vi "Robotics Environment Simulator.vi"() -> ()   [LabVIEW 2015]
doc: "This VI starts and stops the environment simulator and serves as the master VI for your simulation code. Open and run this VI to display the environment simulator, or open the block diagram to view or modify simulation code."
uses:
  <vilib>/Platform/TimedLoop/XDataNode/timing_clust.ctl
  <vilib>/Platform/TimedLoop/XDataNode/nitl_modes.ctl
  <vilib>/Platform/TimedLoop/XDataNode/wakeup.ctl
  <vilib>/Utility/AngleManip/Degrees to Radians (Scalar DBL).vi
  <vilib>/imath/engines/lvmath2/RunTimeEngine/IndexReplace/NIMS M(S,$)=V.vi
  <instcachedir>/0/NIMS M(S,$)=V_260679A9E30142119AFD27BBD2C5FD93.lvgen/NIMS M(S,$)=V_260679A9E30142119AFD27BBD2C5FD93_002.vi
  <vilib>/imathl/engines/lvmath/Functions/Error Handling/Create Error.vi
  <vilib>/imath/engines/lvmath2/RunTimeEngine/IndexReplace/NIMS M(S,S)=S.vi
  <instcachedir>/0/NIMS M(S,S)=S_72298AC072A24B679F5E0C14DB2DD503.lvgen/NIMS M(S,S)=S_72298AC072A24B679F5E0C14DB2DD503_002.vi
  <vilib>/imath/engines/lvmath2/RunTimeEngine/RangeToken/NIMS_Range_R2 - Integer.vi
  <instcachedir>/0/NIMS_Range_R2 - Integer_396D5D4FB869421F9245109A0975AD54.lvgen/NIMS_Range_R2 - Integer_396D5D4FB869421F9245109A0975AD54_000.vi
  <vilib>/imath/engines/lvmath2/RunTimeEngine/CommandStatement/MC_CommandStatement_break.vi
  <vilib>/imath/engines/lvmath2/RunTimeEngine/BuiltInFunctions/mod/NIMS_mod_no_size_check.vi
  <instcachedir>/0/NIMS_mod_no_size_check_5393E3382FD241D281EEB71DA286C65B.lvgen/NIMS_mod_no_size_check_5393E3382FD241D281EEB71DA286C65B_001.vi
  <vilib>/imath/engines/lvmath2/RunTimeEngine/VariableToken/NIMS_VariableToken_CondDefinedDefinedByReplace.vi
  <instcachedir>/0/NIMS_VariableToken_CondDefinedDefinedByReplace_D162CFFC24174562A9FEA619A91E1A56.lvgen/NIMS_VariableToken_CondDefinedDefinedByReplace_D162CFFC24174562A9FEA619A91E1A56_001.vi
  <instcachedir>/0/NIMS M(S,S)=S_72298AC072A24B679F5E0C14DB2DD503.lvgen/NIMS M(S,S)=S_72298AC072A24B679F5E0C14DB2DD503_000.vi
  <vilib>/imath/engines/lvmath2/RunTimeEngine/IndexRead/NIMS M(S,S).vi
  <instcachedir>/0/NIMS M(S,S)_AC51E74150A542F7991B9634C66F3096.lvgen/NIMS M(S,S)_AC51E74150A542F7991B9634C66F3096_000.vi
  <vilib>/imath/engines/lvmath2/RunTimeSupport/NIMS_Error if Not Equal.vi
  <instcachedir>/0/NIMS_Error if Not Equal_7F0D61CE56BF44979916ECA34C78675F.lvgen/NIMS_Error if Not Equal_7F0D61CE56BF44979916ECA34C78675F_000.vi
  <instcachedir>/0/NIMS M(S,S)_AC51E74150A542F7991B9634C66F3096.lvgen/NIMS M(S,S)_AC51E74150A542F7991B9634C66F3096_002.vi
  <vilib>/imath/engines/lvmath2/RunTimeEngine/ErrorHandling/NIMS_Create Error From Enums.vi
  <vilib>/imath/engines/lvmath2/RunTimeEngine/CommandStatement/NIMS_CommandStatement_MaskErr.vi
  <vilib>/imath/engines/lvmath2/RunTimeEngine/VariableToken/NIMS_VariableToken_CondDefined.vi
  <instcachedir>/0/NIMS_VariableToken_CondDefined_FE30D0A1BFB24F098D41DEBABFE96BE1.lvgen/NIMS_VariableToken_CondDefined_FE30D0A1BFB24F098D41DEBABFE96BE1_001.vi
  <vilib>/imath/engines/lvmath2/RunTimeEngine/IndexRead/NIMS M(S,$).vi
  <instcachedir>/0/NIMS M(S,$)_F24F360562DE41D8BE234322A2E15C65.lvgen/NIMS M(S,$)_F24F360562DE41D8BE234322A2E15C65_000.vi
  Documents/LabVIEW Data/MathScriptVIs/MCStatic_35241984432_878391c453101b8ea8a3a082d24a9a1b.vi
  <instcachedir>/0/MCStatic_35241984432_878391c453101b8ea8a3a082d24a9a1b_1C0BCF58ECF54AF19A642F074C09ACBC.lvgen/MCStatic_35241984432_878391c453101b8ea8a3a082d24a9a1b_1C0BCF58ECF54AF19A642F074C09ACBC_000.vi
  <vilib>/imath/engines/lvmath/Functions/Error Handling/MergeErrorsWrapper.vi
  <vilib>/imath/engines/lvmath2/RunTimeEngine/NodeEndStatement/NIMS_NodeEndStatement_Output.vi
  <instcachedir>/0/NIMS_NodeEndStatement_Output_53EC0D466D134D7ABD903AC30B43404B.lvgen/NIMS_NodeEndStatement_Output_53EC0D466D134D7ABD903AC30B43404B_012.vi
  <instcachedir>/0/NIMS_NodeEndStatement_Output_53EC0D466D134D7ABD903AC30B43404B.lvgen/NIMS_NodeEndStatement_Output_53EC0D466D134D7ABD903AC30B43404B_010.vi
  <instcachedir>/0/NIMS_NodeEndStatement_Output_53EC0D466D134D7ABD903AC30B43404B.lvgen/NIMS_NodeEndStatement_Output_53EC0D466D134D7ABD903AC30B43404B_002.vi
  <vilib>/imath/engines/lvmath2/RunTimeEngine/ErrorHandling/NIMS_Finalize Error.vi
  <vilib>/robotics/Steering/Steering Frame/Apply Steering Frame Velocity to Motors.vi
  <instcachedir>/0/NIMS_VariableToken_CondDefined_FE30D0A1BFB24F098D41DEBABFE96BE1.lvgen/NIMS_VariableToken_CondDefined_FE30D0A1BFB24F098D41DEBABFE96BE1_004.vi
  <instcachedir>/0/NIMS_NodeEndStatement_Output_53EC0D466D134D7ABD903AC30B43404B.lvgen/NIMS_NodeEndStatement_Output_53EC0D466D134D7ABD903AC30B43404B_005.vi
  <instcachedir>/0/NIMS_NodeEndStatement_Output_53EC0D466D134D7ABD903AC30B43404B.lvgen/NIMS_NodeEndStatement_Output_53EC0D466D134D7ABD903AC30B43404B_013.vi
  <instcachedir>/0/NIMS_NodeEndStatement_Output_53EC0D466D134D7ABD903AC30B43404B.lvgen/NIMS_NodeEndStatement_Output_53EC0D466D134D7ABD903AC30B43404B_001.vi
  <vilib>/imath/engines/lvmath2/RunTimeEngine/Managers/WorkSpace/UID Generator.vi
  <vilib>/imath/engines/lvmath2/RunTimeEngine/IndexRead/NIMS M($,S).vi
  <instcachedir>/0/NIMS M($,S)_3E5749BBB62E49528D4765A77F1F6D98.lvgen/NIMS M($,S)_3E5749BBB62E49528D4765A77F1F6D98_000.vi
  <vilib>/imath/engines/lvmath2/RunTimeEngine/RunTimeType/NIMS_RunTimeType_From StrictType (excl LVString).vi
  <instcachedir>/0/NIMS_RunTimeType_From StrictType (excl LVString)_EB1C38A9BC5048DA9ABDA8F781E54D21.lvgen/NIMS_RunTimeType_From StrictType (excl LVString)_EB1C38A9BC5048DA9ABDA8F781E54D21_000.vi
  <vilib>/imath/engines/lvmath2/RunTimeEngine/LocalVariableDefStatement/MC_LocalVariableDefStatement_Display.vi
  <vilib>/imath/engines/lvmath2/RunTimeEngine/Managers/SymbolTable/Clear UID.vi
  <vilib>/Platform/TimedLoop/XDataNode/XDataNode.xnode
  Documents/LabVIEW Data/eatbean2.m
  <vilib>/robotics/Starter Kit/2.0/Sim Host Interface/NI_Robotics_Starter Kit Host_Sim_2.0.lvclass
  <vilib>/robotics/Simulator/NI_Robotics_Simulator.lvlib
  <vilib>/Platform/TimedLoop/XDataNode/XDNodeRunTimeDep.lvlib
  <vilib>/robotics/Steering/Steering Frame/NI_Robotics_Steering Frame.lvclass
  <vilib>/robotics/Starter Kit/Host Interface/NI_Robotics_Starter Kit Host.lvclass
  <vilib>/robotics/Utilities/Scan Angles/NI_Robotics_Scan Angles.lvlib
  <vilib>/Utility/AngleManip/NI_AngleManipulation.lvlib
  <vilib>/robotics/Starter Kit/2.0/NI_Robotics_Starter Kit Host_2.0.lvlib
  <vilib>/imath/engines/lvmath2/RunTimeEngine/Managers/SymbolTable/NIMS_WorkSpace.lvlib
panel:
  out "a":dbl[](array[numeric])
  out "b":dbl[](array[numeric])
  out "XY Graph":cluster{"xi":dbl[], "yi":dbl[]}[](graph)
  out "bean":dbl[][](array[numeric])
  in  "stop 3":bool
  out "Sensor Data 2":cluster{"angles (deg)":dbl[], "distances":dbl[]}(graph)
  out "new_angle 2":dbl
  out "new_x 2":dbl
  out "new_y 2":dbl
  out "distances 2":dbl[](array[numeric])
  out "angles 2":dbl[](array[numeric])
  out "v1_next 2":dbl
  out "v2_next 2":dbl
  out "left motor ccw velocity (rad/s) 2":dbl
  out "right motor ccw velocity (rad/s) 2":dbl
  out "headDest":dbl[](array[numeric])
  out "headIndex":i64
  out "headDirect":i32
  in  "stop 2":bool
  out "Sensor Data":cluster{"angles (deg)":dbl[], "distances":dbl[]}(graph)
  out "new_angle":dbl
  out "new_x":dbl
  out "new_y":dbl
  out "distances":dbl[](array[numeric])
  out "angles":dbl[](array[numeric])
  out "v1_next":dbl
  out "v2_next":dbl
  out "left motor ccw velocity (rad/s)":dbl
  out "right motor ccw velocity (rad/s)":dbl
  out "tailIndex":i64
  out "tailDest":dbl[](array[numeric])
  out "tailMoveto":i32
  out "tailDirect":i32
  in  "manifest filename":string="Robotics Environment Simulator.xml"
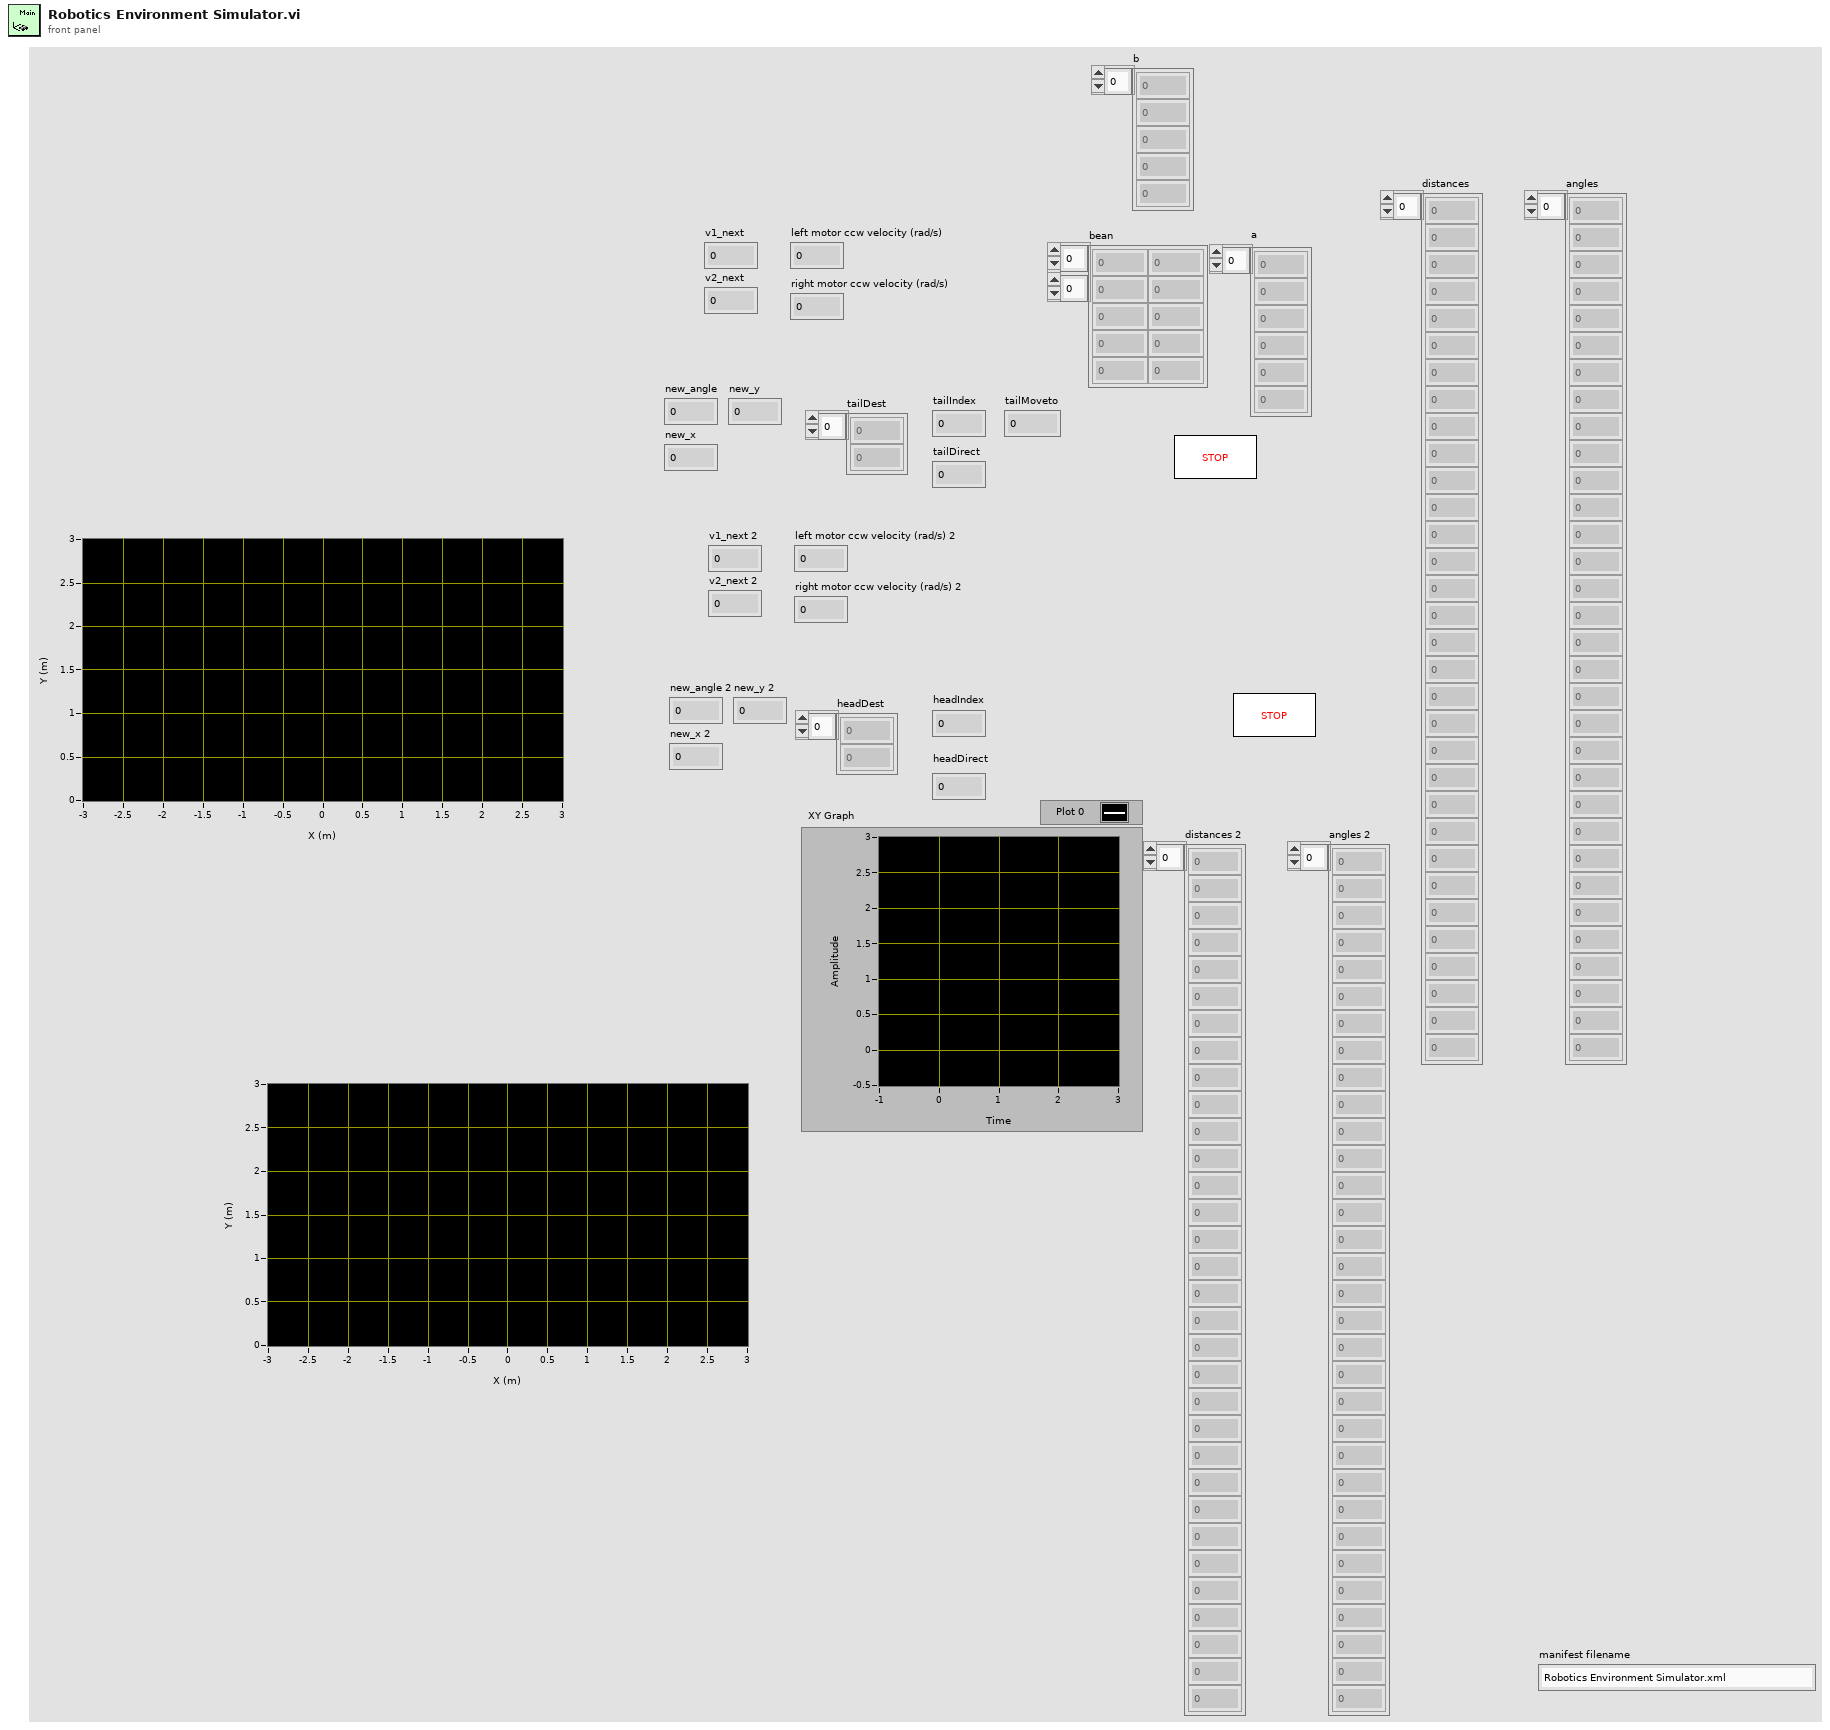
[diagram p1: front panel]
types:
  T1 = typedef "NI_Robotics_Scan Angles.lvlib/Scan Angle Data.ctl" = cluster{"angles":dbl[], "distances":dbl[], "current index":i32, "previous index":i32}
  T2 = typedef "XDNodeRunTimeDep.lvlib/timing_clust.ctl" = cluster{"Expected End [f-1]":u64, "Actual End [f-1]":u64, "Finished Late? [f-1]":bool, "Expected End [i-1]":u64, "Actual End [i-1]":u64, "Finished Late? [i-1]":bool, "Expected Start [i]":u64, "Actual Start [i]":u64, "Expected Start [f]":u64, "Actual Start [f]":u64, "Source Name":string, "Structure Name":string, "Period":i64, "Deadline":i64, "Offset":i64, "Start":i64, "Priority":i32, "Timeout":i32, "Mode":T3, "Wakeup Reason":T4, "Error":errorcluster, "Source Type":string, "Secondary Source Type":string, "Global End Time":u64, "Global Start Time":u64, "Frame Duration":u64, "Iteration Duration":u64, "Assigned CPU":i32, "I/O Scan Engine Mode":u32}
  T3 = typedef "XDNodeRunTimeDep.lvlib/nitl_modes.ctl" = enum32{"No Change", "Process missed periods, maintain original phase", "Discard missed periods, maintain original phase", "Process missed periods, ignore original phase", "Discard missed periods, ignore original phase"}
  T4 = typedef "XDNodeRunTimeDep.lvlib/wakeup.ctl" = enum32{"Normal", "Aborted", "Asynchronous wakeup", "Timing source error", "Timed loop error", "Timeout"}
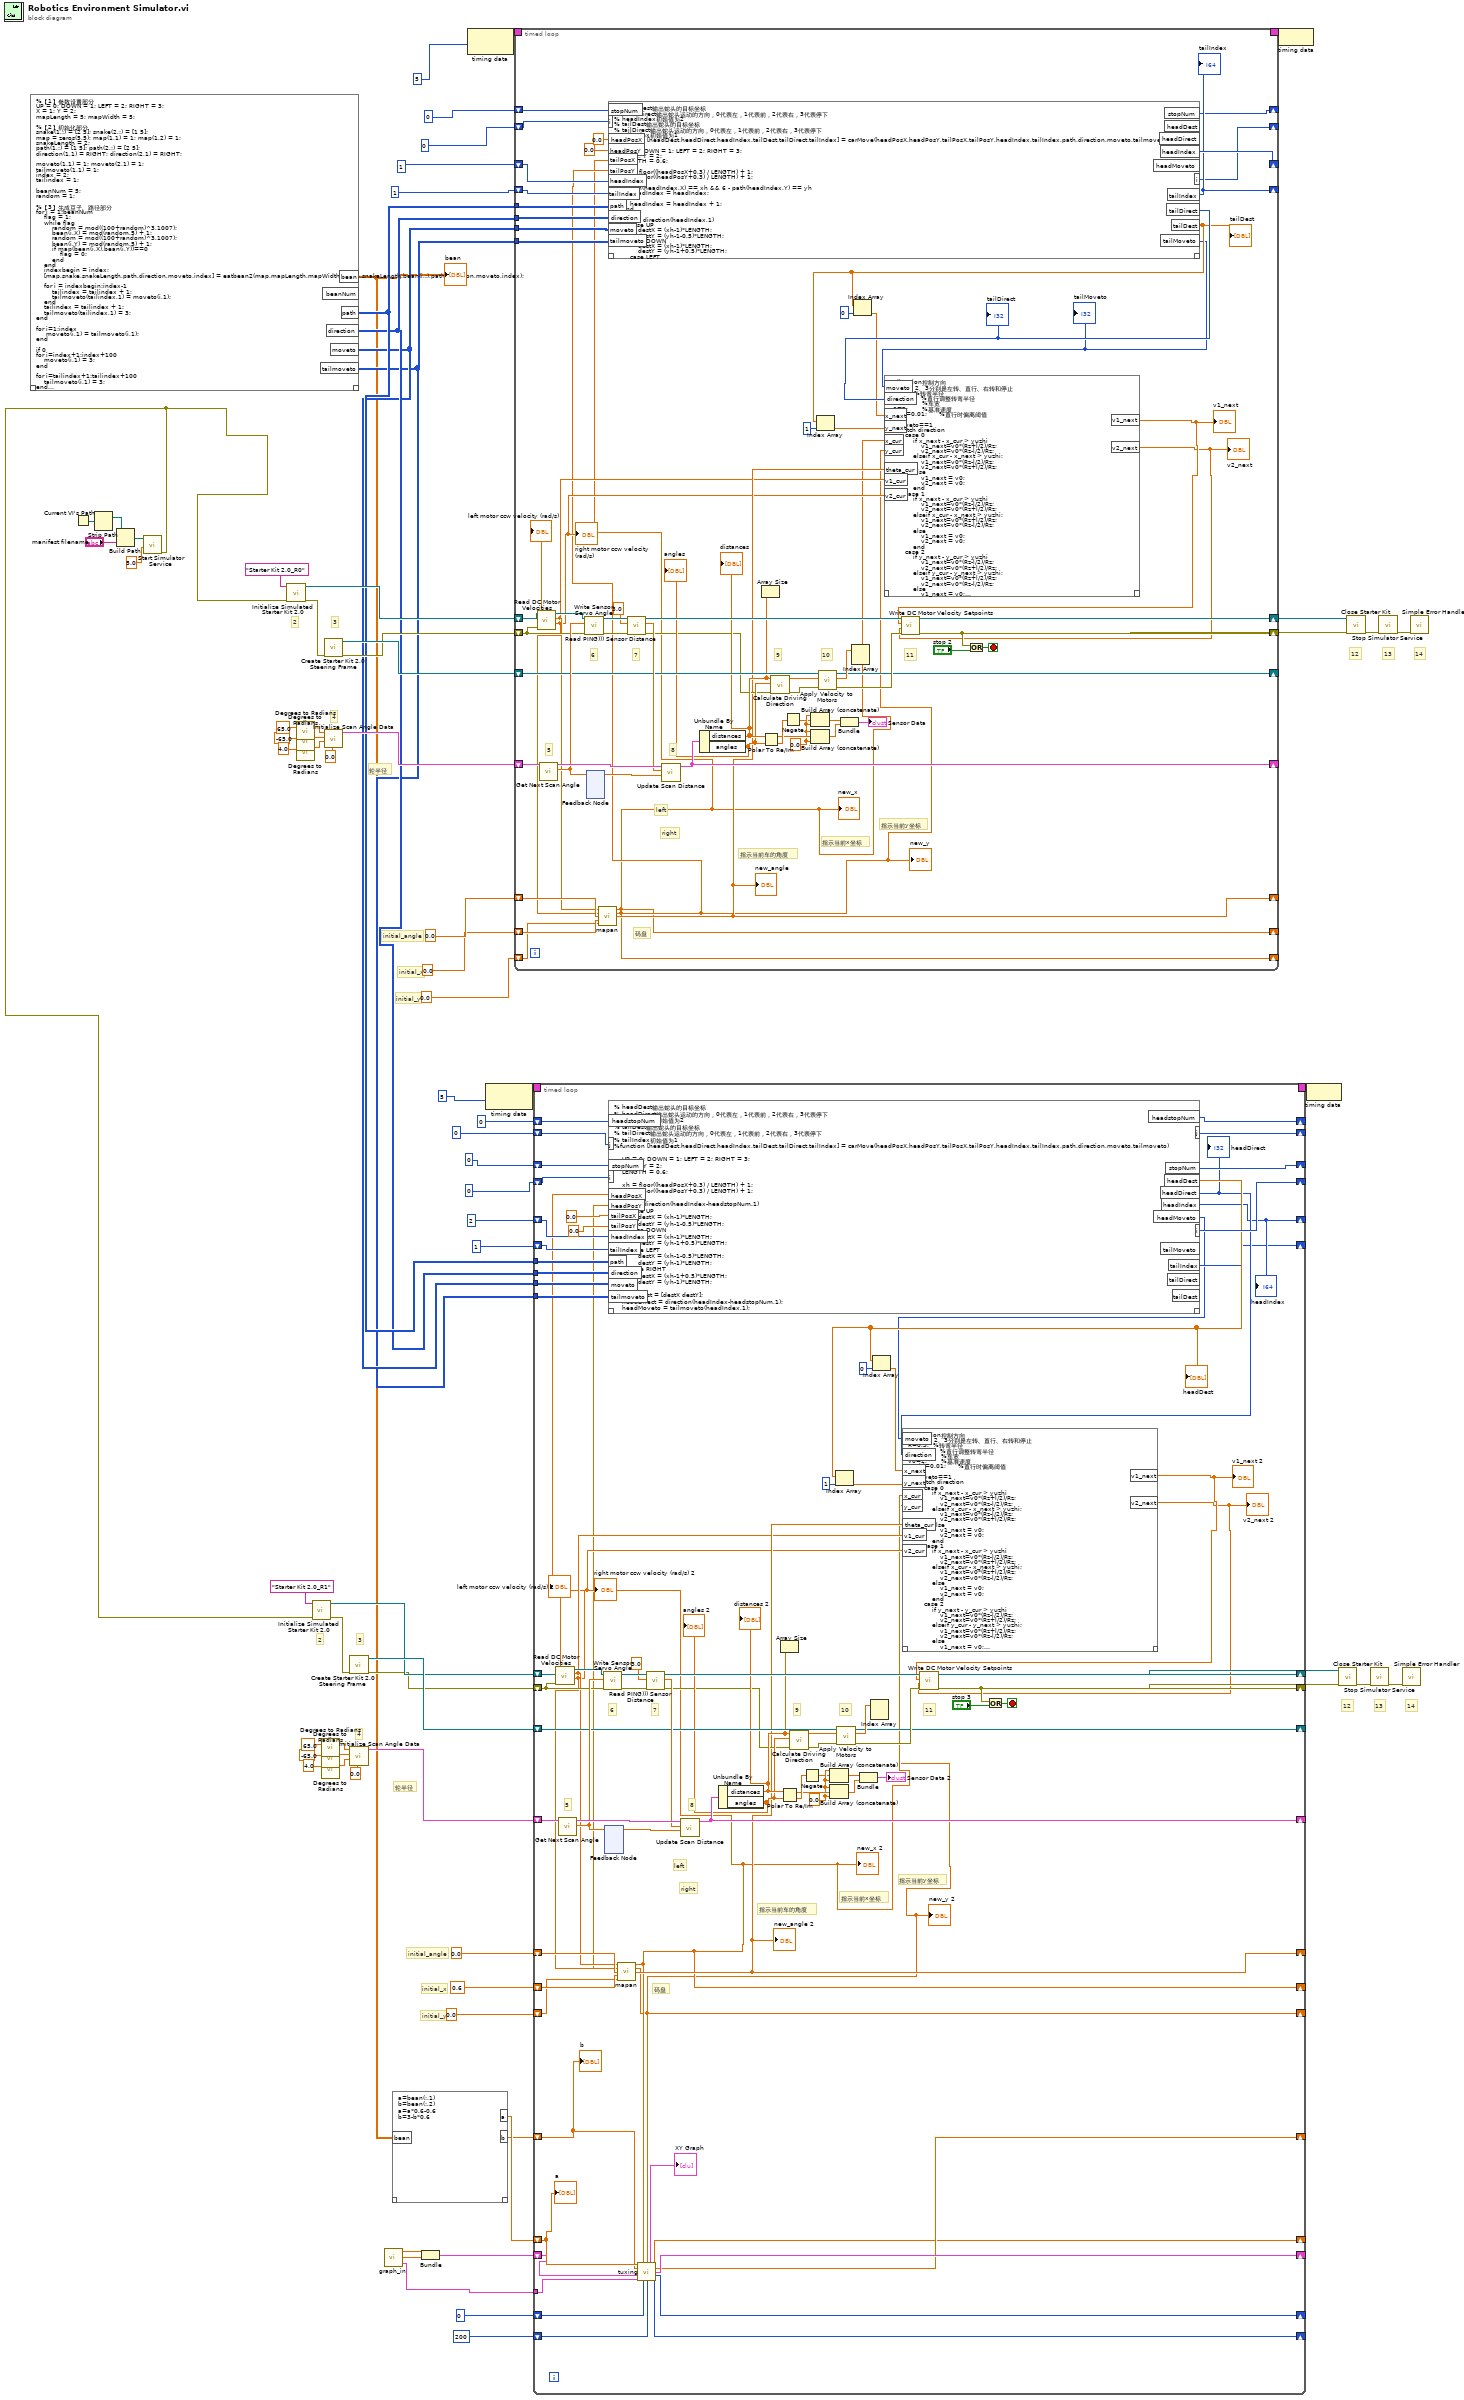
[diagram p0: block diagram]
diagram:
  # "initial_x"
  # "轮半径"
  # "initial_y"
  # "initial_angle"
  # "14"
  # "13"
  # "12"
  # "2"
  # "3"
  # "4"
  # "轮半径"
  # "initial_y"
  # "initial_x"
  # "initial_angle"
  # "14"
  # "13"
  # "12"
  # "2"
  # "3"
  # "4"
  n1 = mathscript code="%【1】参数设置部分\nUP = 0; DOWN = 1; LEFT = 2; RIGHT = 3;\nX = 1; Y = 2;\nmapLength = 5; mapWidth = 5;\n\n%【2】初始化部分\nsnake(1,:) = [2 5]; snake(2,:) = [1 5];\nmap = zeros(5,5); map(1,1) = 1; map(1,2) = 1;\nsnakeLength = 2;\npath(1,:) = [1 5]; path(2,:) = [2 5];\ndirection(1,1) = RIGHT; direction(2,1) = RIGHT;\n    \nmoveto(1,1) = 1; moveto(2,1) = 1;\ntailmoveto(1,1) = 1;\nindex = 2;\ntailindex = 1;\n    \nbeanNum = 5;\nrandom = 1;\n\n%【3】生成豆子、路径部分\nfor i = 1:beanNum\n    flag = 1;\n    while flag\n        random = mod((100+random)^3,1007);\n        bean(i,X) = mod(random,5) + 1;\n        random = mod((100+random)^3,1007);\n        bean(i,Y) = mod(random,5) + 1;\n        if map(bean(i,X),bean(i,Y))==0\n            flag = 0;\n        end\n    end\n    indexbegin = index;\n    [map,snake,snakeLength,path,direction,moveto,index] = eatbean2(map,mapLength,mapWidth,snake,snakeLength,bean(i,:),path,direction,moveto,index);\n    \n    for i = indexbegin:index-1\n        tailindex = tailindex + 1;\n        tailmoveto(tailindex,1) = moveto(i,1);\n    end\n    tailindex = tailindex + 1;\n    tailmoveto(tailindex,1) = 3;\nend\n\nfor i=1:index\n     moveto(i,1) = tailmoveto(i,1);\nend\n\nif 0\nfor i=index+1:index+100\n    moveto(i,1) = 3;\nend\n\nfor i=tailindex+1:tailindex+100\n    tailmoveto(i,1) = 3;\nend\nend"() -> ("bean"=w9:dbl[][], "path"=w16:i32[][], "direction"=w15:i32[][], "moveto"=w14:i32[][], "tailmoveto"=w13:i32[][])  [unwired: 1 in, 2 out]
  "bean" <- w9
  n2 = Current VI's Path() -> (path=w74:path)
  n3 = Strip Path(path=w74) -> (stripped path=w73:path)  [unwired: 1 out]
  n4 = Build Path(base path=w73, name or relative path="manifest filename") -> (appended path=w72:path)
  n5 = call <vilib>:"Start Simulator Service.vi"("step size (ms)"=5.0 ("stepsize(ms)"), "manifest file"=w72) -> ("error out"=w10:errorcluster)  [unwired: 9 in]
  n6 = call <vilib>:"Initialize Simulated Starter Kit 2.0.vi"("error in (no error)"=w10, "robot ID"="Starter Kit 2.0_R0") -> ("error out"=w64:errorcluster, "simulated starter kit host 2.0 out"=w65:refnum<class "NI_Robotics_Starter Kit Host_Sim_2.0.lvclass">)  [unwired: 8 in]
  n7 = call-poly <vilib>:"Degrees to Radians.vi"("angle (deg)"=65.0 ("max angle")) -> ("angle (rad)"=w60:dbl)  [unwired: 2 in]
  n8 = call-poly <vilib>:"Degrees to Radians.vi"("angle (deg)"=-65.0 ("min angle")) -> ("angle (rad)"=w56:dbl)  [unwired: 2 in]
  n9 = call-poly <vilib>:"Degrees to Radians.vi"("angle (deg)"=4.0 ("scan angle")) -> ("angle (rad)"=w57:dbl)  [unwired: 2 in]
  n10 = call <vilib>:"Initialize Simulated Starter Kit 2.0.vi"("error in (no error)"=w10, "robot ID"="Starter Kit 2.0_R1") -> ("error out"=w39:errorcluster, "simulated starter kit host 2.0 out"=w40:refnum<class "NI_Robotics_Starter Kit Host_Sim_2.0.lvclass">)  [unwired: 8 in]
  n11 = call-poly <vilib>:"Degrees to Radians.vi"("angle (deg)"=65.0 ("max angle")) -> ("angle (rad)"=w35:dbl)  [unwired: 2 in]
  n12 = call-poly <vilib>:"Degrees to Radians.vi"("angle (deg)"=-65.0 ("min angle")) -> ("angle (rad)"=w31:dbl)  [unwired: 2 in]
  n13 = call-poly <vilib>:"Degrees to Radians.vi"("angle (deg)"=4.0 ("scan angle")) -> ("angle (rad)"=w32:dbl)  [unwired: 2 in]
  n14 = call <vilib>:"Create Starter Kit 2.0 Steering Frame.vi"("error in (no error)"=w64) -> ("error out"=w54:errorcluster, "starter kit differential steering frame"=w66:refnum<class "NI_Robotics_Differential Steering Frame.lvclass">)  [unwired: 9 in]
  n15 = call <vilib>:"Initialize Scan Angle Data.vi"("initial angle (0)"=0.0, "scan angle"=w57, "min angle"=w56, "max angle"=w60) -> ("scan angles"=w55:T1)  [unwired: 6 in, 1 out]
  n16 = call <vilib>:"Create Starter Kit 2.0 Steering Frame.vi"("error in (no error)"=w39) -> ("error out"=w29:errorcluster, "starter kit differential steering frame"=w41:refnum<class "NI_Robotics_Differential Steering Frame.lvclass">)  [unwired: 9 in]
  n17 = call <vilib>:"Initialize Scan Angle Data.vi"("initial angle (0)"=0.0, "scan angle"=w32, "min angle"=w31, "max angle"=w35) -> ("scan angles"=w30:T1)  [unwired: 6 in, 1 out]
  n18 = call "graph_in.vi"() -> ("map"=w3:cluster{"x":dbl[], "y":dbl[]}, "y0"=w5:dbl[], "x0"=w6:dbl[])
  n19 = mathscript code="a=bean(:,1)\nb=bean(:,2)\na=a*0.6-0.6\nb=3-b*0.6"("bean"=w9) -> ("a"=w8:dbl[], "b"=w7:dbl[])  [unwired: 1 in, 1 out]
  n20 = Bundle("x0"=w6, "y0"=w5) -> (w4:cluster{"x0":dbl[], "y0":dbl[]})  [unwired: 1 in]
  n21 = node-c288(i64 5 ("Period")) -> (w70:T2)
  n22 = node-c288(i64 5 ("Period")) -> (w68:T2)
  n23 = timed-loop {
    shift-right: [w124] -> w63
    shift-left: w65 -> [w111]
    shift-right: [w113] -> w62
    shift-left: w54 -> [w112]
    shift-right: [w126] -> _
    shift-left: w66 -> [w127]
    timing: w70 -> [_]
    timing-out: [_] -> w69
    shift-right: [w123] -> _
    shift-left: w55 -> [w128]
    shift-right: [w103] -> _
    shift-left: 0.0 -> [w106]
    shift-right: [w89] -> _
    shift-left: 0.0 -> [w105]
    shift-right: [w90] -> _
    shift-left: 0.0 -> [w104]
    tunnel: w16 -> [w100]
    tunnel: w15 -> [w97]
    tunnel: w14 -> [w99]
    tunnel: w13 -> [w98]
    shift-right: [w95] -> _
    shift-left: i64 1 ("Period") -> [w96]
    shift-right: [w94] -> _
    shift-left: i64 1 ("Period") -> [w93]
    shift-right: [w83] -> _
    shift-left: i64 0 ("Period") -> [w84]
    shift-right: [w81] -> _
    shift-left: i64 0 ("Period") -> [w82]
    stop <- w125 stop-if-true
    w119 = 0.0 ("element")
    # "指示当前y坐标"
    # "指示当前x坐标"
    # "指示当前车的角度"
    # "码盘"
    # "right"
    # "left"
    # "7"
    # "6"
    # "11"
    # "10"
    # "9"
    # "8"
    # "5"
    n24 = call <vilib>:"Read DC Motor Velocities.vi"("error in (no error)"=w112, "starter kit host in"=w111) -> ("right motor ccw velocity (rad/s)"=w101:dbl, "left motor ccw velocity (rad/s)"=w102:dbl, "starter kit host out"=w110:refnum<class "NI_Robotics_Starter Kit Host_Sim_2.0.lvclass">)  [unwired: 6 in, 1 out]
    "left motor ccw velocity (rad/s)" <- w102
    "right motor ccw velocity (rad/s)" <- w101
    n25 = call <vilib>:"Get Next Scan Angle.vi"("scan angles in"=w128) -> ("new angle"=w135:dbl, "scan angles out"=w138:T1)  [unwired: 9 in]
    n26 = call <vilib>:"Write Sensor Servo Angle.vi"("error in (no error)"=w112, "ccw servo angle (rad)"=w135, "starter kit host in"=w110) -> ("error out"=w132:errorcluster, "starter kit host out"=w133:refnum<class "NI_Robotics_Starter Kit Host_Sim_2.0.lvclass">)  [unwired: 7 in]
    n27 = feedback #1() -> (w137:dbl)  [unwired: 1 in]
    n28 = feedback-in #1(w135) -> ()
    n29 = call "mapan.vi"("lwf"=w102, "rwf"=w101, "direct"=w106, "xposit"=w105, "yposit"=w104) -> ("xposit 2"=w89:dbl, "yposit 2"=w90:dbl, "direct 2"=w103:dbl)  [unwired: 8 in]
    "new_angle" <- w103
    "new_x" <- w89
    "new_y" <- w90
    n30 = mathscript code="% headDest输出蛇头的目标坐标\n% headDirect输出蛇头运动的方向，0代表左，1代表前，2代表右，3代表停下\n% headIndex初始值为2\n% tailDest输出蛇头的目标坐标\n% tailDirect输出蛇头运动的方向，0代表左，1代表前，2代表右，3代表停下\n% tailIndex初始值为1\n%function [headDest,headDirect,headIndex,tailDest,tailDirect,tailIndex] = carMove(headPosX,headPosY,tailPosX,tailPosY,headIndex,tailIndex,path,direction,moveto,tailmoveto)\n\nUP = 0; DOWN = 1; LEFT = 2; RIGHT = 3;\n    X = 1; Y = 2;\n    LENGTH = 0.6;\n    \n    xh = floor((headPosX+0.3) / LENGTH) + 1;\n    yh = floor((headPosY+0.3) / LENGTH) + 1;\n    \n    if path(headIndex,X) == xh && 6 - path(headIndex,Y) == yh\n        headIndex = headIndex;\n    else\n        headIndex = headIndex + 1;\n    end\n    \n    switch direction(headIndex,1)\n        case UP\n            destX = (xh-1)*LENGTH;\n            destY = (yh-1-0.5)*LENGTH;\n        case DOWN\n            destX = (xh-1)*LENGTH;\n            destY = (yh-1+0.5)*LENGTH;\n        case LEFT\n            destX = (xh-1-0.5)*LENGTH;\n            destY = (yh-1)*LENGTH;\n        case RIGHT\n            destX = (xh-1+0.5)*LENGTH;\n            destY = (yh-1)*LENGTH;\n    end\n    headDest = [destX destY];\n    headDirect = direction(headIndex,1);\n    headMoveto = moveto(headIndex,1);\n    \n    xt = floor((tailPosX+0.3) / LENGTH) + 1;\n    yt = floor((tailPosY+0.3) / LENGTH) + 1;\n\n    switch direction(tailIndex-stopNum,1)\n        case UP\n            destX = (xt-1)*LENGTH;\n            destY = (yt-1-0.5)*LENGTH;\n        case DOWN\n            destX = (xt-1)*LENGTH;\n            destY = (yt-1+0.5)*LENGTH;\n        case LEFT\n            destX = (xt-1-0.5)*LENGTH;\n            destY = (yt-1)*LENGTH;\n        case RIGHT\n            destX = (xt-1+0.5)*LENGTH;\n            destY = (yt-1)*LENGTH;\n    end\n    tailDest = [destX destY];\n    tailDirect = direction(tailIndex-stopNum,1);\n    tailMoveto = tailmoveto(tailIndex,1);\n\n    if tailMoveto==3\n        if i<1200\n            i = i + 1;\n            tailIndex = tailIndex;\n        else\n            i = 0;\n            tailIndex = tailIndex + 1;\n            stopNum = stopNum + 1;\n        end\n    elseif path(tailIndex-stopNum,X) == xt && (6 - path(tailIndex-stopNum,Y) == yt)\n        tailIndex = tailIndex;\n    else\n        tailIndex = tailIndex + 1;\n    end"("headPosX"=0.0, "headPosY"=0.0, "tailPosX"=w89, "tailPosY"=w90, "headIndex"=w96, "tailIndex"=w93, "path"=w100, "direction"=w97, "moveto"=w99, "tailmoveto"=w98, "i"=w84, "stopNum"=w82) -> ("headIndex"=w95:i64, "tailIndex"=w94:i64, "tailDirect"=w88:i32, "tailDest"=w87:dbl[], "i"=w83:i64, "stopNum"=w81:i64, "tailMoveto"=w76:i32)  [unwired: 1 in, 4 out]
    "tailIndex" <- w94
    "tailDest" <- w87
    "tailMoveto" <- w76
    "tailDirect" <- w88
    n31 = call <vilib>:"Read PING))) Sensor Distance.vi"("error in (no error)"=w132, "default distance (NaN)"=3.0, "starter kit host in"=w133) -> ("error out"=w107:errorcluster, "distance (m)"=w134:dbl, "starter kit host out"=w131:refnum<class "NI_Robotics_Starter Kit Host_Sim_2.0.lvclass">)  [unwired: 5 in, 1 out]
    n32 = call <vilib>:"Update Scan Distance.vi"("scan angle"=w137, "new scan distance"=w134, "scan angles in"=w138) -> ("scan angles out"=w123:T1)  [unwired: 8 in]
    n33 = Unbundle By Name(w123) -> ("distances"=w109:dbl[], "angles"=w108:dbl[])
    "distances" <- w109
    "angles" <- w108
    n34 = Array Size(array=w109) -> ()  [unwired: 1 out]
    n35 = Polar To Re/Im(2:w108, 3:w109) -> (0:w122:dbl[], 1:w121:dbl[])
    n36 = call "Calculate Driving Direction.vi"("error in (no error)"=w107, "obstacle angles (rad)"=w108, "obstacle distances (m)"=w109) -> ("error out"=w114:errorcluster, "steering frame velocity"=w115:dbl[])  [unwired: 7 in]
    n37 = Negate(x=w122) -> (-x=w117:dbl[])
    n38 = Build Array (concatenate)(w119, w117, w119) -> (w118:dbl[])
    n39 = Build Array (concatenate)(w119, w121, w119) -> (w120:dbl[])
    n40 = Index Array(array=w87, index=1) -> (element=w79:dbl)
    n41 = call-poly <vilib>:"Apply Velocity to Motors.vi"("error in (no error)"=w114, "steering frame velocity"=w115, "steering frame in"=w127) -> ("error out"=w130:errorcluster, "ccw motor velocity setpoints"=w136:dbl[], "steering frame out"=w126:refnum<class "NI_Robotics_Differential Steering Frame.lvclass">)  [unwired: 4 in, 2 out]
    n42 = Bundle(w118, w120) -> (→"Sensor Data":cluster{dbl[], dbl[]})  [unwired: 1 in]
    n43 = Index Array(array=w136) -> ()  [unwired: 2 in, 2 out]
    n44 = Index Array(array=w87, index=0) -> (element=w80:dbl)
    n45 = mathscript code="%direction控制方向\n%0、1、2、3分别是左转、直行、右转和停止\nR=0.3;  %转弯半径\nRz=1.5;    %直行调整转弯半径\nl=0.36;     %车宽\nv0=2;       %基准速度\nyuzhi=0.01;      %直行时偏离阈值\n\nif moveto==1\n    switch direction\n        case 0\n            if x_next - x_cur > yuzhi\n                v1_next=v0*(Rz+l/2)/Rz;\n                v2_next=v0*(Rz-l/2)/Rz;\n            elseif x_cur - x_next > yuzhi;\n                v1_next=v0*(Rz-l/2)/Rz;\n                v2_next=v0*(Rz+l/2)/Rz;\n            else\n                v1_next = v0;\n                v2_next = v0;\n            end\n        case 1\n            if x_next - x_cur > yuzhi\n                v1_next=v0*(Rz-l/2)/Rz;\n                v2_next=v0*(Rz+l/2)/Rz;\n            elseif x_cur - x_next > yuzhi;\n                v1_next=v0*(Rz+l/2)/Rz;\n                v2_next=v0*(Rz-l/2)/Rz;\n            else\n                v1_next = v0;\n                v2_next = v0;\n            end\n        case 2\n            if y_next - y_cur > yuzhi\n                v1_next=v0*(Rz-l/2)/Rz;\n                v2_next=v0*(Rz+l/2)/Rz;\n            elseif y_cur - y_next > yuzhi;\n                v1_next=v0*(Rz+l/2)/Rz;\n                v2_next=v0*(Rz-l/2)/Rz;\n            else\n                v1_next = v0;\n                v2_next = v0;\n            end\n        case 3\n            if y_next - y_cur > yuzhi\n                v1_next=v0*(Rz+l/2)/Rz;\n                v2_next=v0*(Rz-l/2)/Rz;\n            elseif y_cur - y_next > yuzhi;\n                v1_next=v0*(Rz-l/2)/Rz;\n                v2_next=v0*(Rz+l/2)/Rz;\n            else\n                v1_next = v0;\n                v2_next = v0;\n            end\n    end\nelseif moveto==0\n    v1_next=v0*(R-l/2)/R;\n    v2_next=v0*(R+l/2)/R;\nelseif moveto==2\n    v1_next=v0*(R+l/2)/R;\n    v2_next=v0*(R-l/2)/R;\nelse\n    if v1_cur>0.8 && v2_cur>0.8\n        v1_next=v1_cur-0.5;\n        v2_next=v2_cur-0.5;\n    else\n        v1_next=0;\n        v2_next=0;\n    end\nend\nv2_next=-v2_next;"("x_next"=w80, "y_next"=w79, "x_cur"=w89, "y_cur"=w90, "theta_cur"=w103, "v1_cur"=w102, "v2_cur"=w101, "direction"=w88, "moveto"=w76) -> ("v1_next"=w78:dbl, "v2_next"=w77:dbl)  [unwired: 1 in, 1 out]
    "v1_next" <- w78
    "v2_next" <- w77
    n46 = call <vilib>:"Write DC Motor Velocity Setpoints.vi"("error in (no error)"=w130, "right motor ccw velocity (rad/s)"=w77, "left motor ccw velocity (rad/s)"=w78, "starter kit host in"=w131) -> ("error out"=w113:errorcluster, "starter kit host out"=w124:refnum<class "NI_Robotics_Starter Kit Host_Sim_2.0.lvclass">)  [unwired: 6 in]
    n47 = Or(x=w113, y="stop 2") -> (x .or. y?=w125:bool)
  }
  n48 = timed-loop {
    shift-right: [w1967] -> w38
    shift-left: w40 -> [w1954]
    shift-right: [w1956] -> w37
    shift-left: w29 -> [w1955]
    shift-right: [w1969] -> _
    shift-left: w41 -> [w1970]
    timing: w68 -> [_]
    timing-out: [_] -> w67
    shift-right: [w1966] -> _
    shift-left: w30 -> [w1971]
    shift-right: [w1946] -> _
    shift-left: 0.0 -> [w1949]
    shift-right: [w1909] -> _
    shift-left: 0.6 -> [w1948]
    shift-right: [w1908] -> _
    shift-left: 0.0 -> [w1947]
    tunnel: w16 -> [w1943]
    tunnel: w15 -> [w1940]
    tunnel: w14 -> [w1942]
    tunnel: w13 -> [w1941]
    shift-right: [w1923] -> _
    shift-left: i64 2 ("Period") -> [w1939]
    shift-right: [w1922] -> _
    shift-left: i64 1 ("Period") -> [w1938]
    shift-right: [w1934] -> _
    shift-left: i64 0 ("Period") -> [w1935]
    shift-right: [w1932] -> _
    shift-left: i64 0 ("Period") -> [w1933]
    shift-right: [w1918] -> _
    shift-left: i64 0 ("Period") -> [w1920]
    shift-right: [w1917] -> _
    shift-left: i64 0 ("Period") -> [w1919]
    tunnel: w3 -> [w1913]
    shift-right: [w1907] -> _
    shift-left: 0 -> [w1912]
    shift-right: [w1906] -> _
    shift-left: 200 -> [w1911]
    shift-right: [w1903] -> _
    shift-left: w8 -> [w1916]
    shift-right: [w1904] -> _
    shift-left: w7 -> [w1915]
    shift-right: [w1905] -> _
    shift-left: w4 -> [w1914]
    stop <- w1968 stop-if-true
    w1962 = 0.0 ("element")
    # "指示当前y坐标"
    # "指示当前x坐标"
    # "指示当前车的角度"
    # "码盘"
    # "right"
    # "left"
    # "7"
    # "6"
    # "11"
    # "10"
    # "9"
    # "8"
    # "5"
    n49 = call <vilib>:"Read DC Motor Velocities.vi"("error in (no error)"=w1955, "starter kit host in"=w1954) -> ("right motor ccw velocity (rad/s)"=w1944:dbl, "left motor ccw velocity (rad/s)"=w1945:dbl, "starter kit host out"=w1953:refnum<class "NI_Robotics_Starter Kit Host_Sim_2.0.lvclass">)  [unwired: 6 in, 1 out]
    "left motor ccw velocity (rad/s) 2" <- w1945
    "right motor ccw velocity (rad/s) 2" <- w1944
    n50 = call <vilib>:"Get Next Scan Angle.vi"("scan angles in"=w1971) -> ("new angle"=w1978:dbl, "scan angles out"=w1981:T1)  [unwired: 9 in]
    n51 = call <vilib>:"Write Sensor Servo Angle.vi"("error in (no error)"=w1955, "ccw servo angle (rad)"=w1978, "starter kit host in"=w1953) -> ("error out"=w1975:errorcluster, "starter kit host out"=w1976:refnum<class "NI_Robotics_Starter Kit Host_Sim_2.0.lvclass">)  [unwired: 7 in]
    n52 = feedback #2() -> (w1980:dbl)  [unwired: 1 in]
    n53 = feedback-in #2(w1978) -> ()
    n54 = call "mapan.vi"("lwf"=w1945, "rwf"=w1944, "direct"=w1949, "xposit"=w1948, "yposit"=w1947) -> ("xposit 2"=w1909:dbl, "yposit 2"=w1908:dbl, "direct 2"=w1946:dbl)  [unwired: 8 in]
    "new_angle 2" <- w1946
    "new_x 2" <- w1909
    "new_y 2" <- w1908
    n55 = mathscript code="% headDest输出蛇头的目标坐标\n% headDirect输出蛇头运动的方向，0代表左，1代表前，2代表右，3代表停下\n% headIndex初始值为2\n% tailDest输出蛇头的目标坐标\n% tailDirect输出蛇头运动的方向，0代表左，1代表前，2代表右，3代表停下\n% tailIndex初始值为1\n%function [headDest,headDirect,headIndex,tailDest,tailDirect,tailIndex] = carMove(headPosX,headPosY,tailPosX,tailPosY,headIndex,tailIndex,path,direction,moveto,tailmoveto)\n\n    UP = 0; DOWN = 1; LEFT = 2; RIGHT = 3;\n    X = 1; Y = 2;\n    LENGTH = 0.6;\n    \n    xh = floor((headPosX+0.3) / LENGTH) + 1;\n    yh = floor((headPosY+0.3) / LENGTH) + 1;\n    \n    switch direction(headIndex-headstopNum,1)\n        case UP\n            destX = (xh-1)*LENGTH;\n            destY = (yh-1-0.5)*LENGTH;\n        case DOWN\n            destX = (xh-1)*LENGTH;\n            destY = (yh-1+0.5)*LENGTH;\n        case LEFT\n            destX = (xh-1-0.5)*LENGTH;\n            destY = (yh-1)*LENGTH;\n        case RIGHT\n            destX = (xh-1+0.5)*LENGTH;\n            destY = (yh-1)*LENGTH;\n    end\n    headDest = [destX destY];\n    headDirect = direction(headIndex-headstopNum,1);\n    headMoveto = tailmoveto(headIndex,1);\n    \n    if headMoveto==3\n        if j<150\n            j = j + 1;\n            headIndex = headIndex;\n        else\n            j = 0;\n            headIndex = headIndex + 1;\n            headstopNum = headstopNum + 1;\n        end\n    elseif path(headIndex-headstopNum,X) == xh && (6 - path(headIndex-headstopNum,Y) == yh)\n        headIndex = headIndex;\n    else\n        headIndex = headIndex + 1;\n    end\n\n    xt = floor((tailPosX+0.3) / LENGTH) + 1;\n    yt = floor((tailPosY+0.3) / LENGTH) + 1;\n\n    switch direction(tailIndex-stopNum,1)\n        case UP\n            destX = (xt-1)*LENGTH;\n            destY = (yt-1-0.5)*LENGTH;\n        case DOWN\n            destX = (xt-1)*LENGTH;\n            destY = (yt-1+0.5)*LENGTH;\n        case LEFT\n            destX = (xt-1-0.5)*LENGTH;\n            destY = (yt-1)*LENGTH;\n        case RIGHT\n            destX = (xt-1+0.5)*LENGTH;\n            destY = (yt-1)*LENGTH;\n    end\n    tailDest = [destX destY];\n    tailDirect = direction(tailIndex-stopNum,1);\n    tailMoveto = tailmoveto(tailIndex,1);\n\n    if tailMoveto==3\n        if i<1200\n            i = i + 1;\n            tailIndex = tailIndex;\n        else\n            i = 0;\n            tailIndex = tailIndex + 1;\n            stopNum = stopNum + 1;\n        end\n    elseif path(tailIndex-stopNum,X) == xt && (6 - path(tailIndex-stopNum,Y) == yt)\n        tailIndex = tailIndex;\n    else\n        tailIndex = tailIndex + 1;\n    end"("headPosX"=w1909, "headPosY"=w1908, "tailPosX"=0.0, "tailPosY"=0.0 ("tailPosX"), "headIndex"=w1939, "tailIndex"=w1938, "path"=w1943, "direction"=w1940, "moveto"=w1942, "tailmoveto"=w1941, "i"=w1935, "stopNum"=w1933, "j"=w1920, "headstopNum"=w1919) -> ("headIndex"=w1923:i64, "tailIndex"=w1922:i64, "headDirect"=w1927:i32, "headDest"=w1929:dbl[], "i"=w1934:i64, "stopNum"=w1932:i64, "headMoveto"=w1921:i32, "j"=w1918:i64, "headstopNum"=w1917:i64)  [unwired: 1 in, 4 out]
    "headDest" <- w1929
    "headIndex" <- w1923
    "headDirect" <- w1927
    n56 = call "tuxing.vi"("bean_x"=w1916, "xnew"=w1909, "ynew"=w1908, "bean_y"=w1915, "xy_in"=w1914, "map_in"=w1913, "n1"=w1912, "n2"=w1911) -> ("XY Graph"=→"XY Graph":cluster{"xi":dbl[], "yi":dbl[]}[], "a"=w1903:dbl[], "b"=w1904:dbl[], "pos_o"=w1905:cluster{"xo":dbl[], "yo":dbl[]}, "n1 2"=w1907:i32, "n2 2"=w1906:i32)  [unwired: 2 in]
    n57 = call <vilib>:"Read PING))) Sensor Distance.vi"("error in (no error)"=w1975, "default distance (NaN)"=3.0, "starter kit host in"=w1976) -> ("error out"=w1950:errorcluster, "distance (m)"=w1977:dbl, "starter kit host out"=w1974:refnum<class "NI_Robotics_Starter Kit Host_Sim_2.0.lvclass">)  [unwired: 5 in, 1 out]
    n58 = call <vilib>:"Update Scan Distance.vi"("scan angle"=w1980, "new scan distance"=w1977, "scan angles in"=w1981) -> ("scan angles out"=w1966:T1)  [unwired: 8 in]
    n59 = Unbundle By Name(w1966) -> ("distances"=w1952:dbl[], "angles"=w1951:dbl[])
    "distances 2" <- w1952
    "angles 2" <- w1951
    n60 = Array Size(array=w1952) -> ()  [unwired: 1 out]
    n61 = Polar To Re/Im(2:w1951, 3:w1952) -> (0:w1965:dbl[], 1:w1964:dbl[])
    n62 = call "Calculate Driving Direction.vi"("error in (no error)"=w1950, "obstacle angles (rad)"=w1951, "obstacle distances (m)"=w1952) -> ("error out"=w1957:errorcluster, "steering frame velocity"=w1958:dbl[])  [unwired: 7 in]
    n63 = Negate(x=w1965) -> (-x=w1960:dbl[])
    n64 = Build Array (concatenate)(w1962, w1960, w1962) -> (w1961:dbl[])
    n65 = Build Array (concatenate)(w1962, w1964, w1962) -> (w1963:dbl[])
    n66 = Index Array(array=w1929, index=1) -> (element=w1930:dbl)
    n67 = call-poly <vilib>:"Apply Velocity to Motors.vi"("error in (no error)"=w1957, "steering frame velocity"=w1958, "steering frame in"=w1970) -> ("error out"=w1973:errorcluster, "ccw motor velocity setpoints"=w1979:dbl[], "steering frame out"=w1969:refnum<class "NI_Robotics_Differential Steering Frame.lvclass">)  [unwired: 4 in, 2 out]
    n68 = Bundle(w1961, w1963) -> (→"Sensor Data 2":cluster{dbl[], dbl[]})  [unwired: 1 in]
    n69 = Index Array(array=w1979) -> ()  [unwired: 2 in, 2 out]
    n70 = Index Array(array=w1929, index=0) -> (element=w1931:dbl)
    n71 = mathscript code="%direction控制方向\n%0、1、2、3分别是左转、直行、右转和停止\nR=0.3;  %转弯半径\nRz=1.5;    %直行调整转弯半径\nl=0.36;     %车宽\nv0=2;       %基准速度\nyuzhi=0.01;      %直行时偏离阈值\n\nif moveto==1\n    switch direction\n        case 0\n            if x_next - x_cur > yuzhi\n                v1_next=v0*(Rz+l/2)/Rz;\n                v2_next=v0*(Rz-l/2)/Rz;\n            elseif x_cur - x_next > yuzhi;\n                v1_next=v0*(Rz-l/2)/Rz;\n                v2_next=v0*(Rz+l/2)/Rz;\n            else\n                v1_next = v0;\n                v2_next = v0;\n            end\n        case 1\n            if x_next - x_cur > yuzhi\n                v1_next=v0*(Rz-l/2)/Rz;\n                v2_next=v0*(Rz+l/2)/Rz;\n            elseif x_cur - x_next > yuzhi;\n                v1_next=v0*(Rz+l/2)/Rz;\n                v2_next=v0*(Rz-l/2)/Rz;\n            else\n                v1_next = v0;\n                v2_next = v0;\n            end\n        case 2\n            if y_next - y_cur > yuzhi\n                v1_next=v0*(Rz-l/2)/Rz;\n                v2_next=v0*(Rz+l/2)/Rz;\n            elseif y_cur - y_next > yuzhi;\n                v1_next=v0*(Rz+l/2)/Rz;\n                v2_next=v0*(Rz-l/2)/Rz;\n            else\n                v1_next = v0;\n                v2_next = v0;\n            end\n        case 3\n            if y_next - y_cur > yuzhi\n                v1_next=v0*(Rz+l/2)/Rz;\n                v2_next=v0*(Rz-l/2)/Rz;\n            elseif y_cur - y_next > yuzhi;\n                v1_next=v0*(Rz-l/2)/Rz;\n                v2_next=v0*(Rz+l/2)/Rz;\n            else\n                v1_next = v0;\n                v2_next = v0;\n            end\n    end\nelseif moveto==0\n    v1_next=v0*(R-l/2)/R;\n    v2_next=v0*(R+l/2)/R;\nelseif moveto==2\n    v1_next=v0*(R+l/2)/R;\n    v2_next=v0*(R-l/2)/R;\nelse\n    if v1_cur>0.8 && v2_cur>0.8\n        v1_next=v1_cur-0.5;\n        v2_next=v2_cur-0.5;\n    else\n        v1_next=0;\n        v2_next=0;\n    end\nend\nv2_next=-v2_next;"("x_next"=w1931, "y_next"=w1930, "x_cur"=w1909, "y_cur"=w1908, "theta_cur"=w1946, "v1_cur"=w1945, "v2_cur"=w1944, "direction"=w1927, "moveto"=w1921) -> ("v1_next"=w1925:dbl, "v2_next"=w1924:dbl)  [unwired: 1 in, 1 out]
    "v1_next 2" <- w1925
    "v2_next 2" <- w1924
    n72 = call <vilib>:"Write DC Motor Velocity Setpoints.vi"("error in (no error)"=w1973, "right motor ccw velocity (rad/s)"=w1924, "left motor ccw velocity (rad/s)"=w1925, "starter kit host in"=w1974) -> ("error out"=w1956:errorcluster, "starter kit host out"=w1967:refnum<class "NI_Robotics_Starter Kit Host_Sim_2.0.lvclass">)  [unwired: 6 in]
    n73 = Or(x=w1956, y="stop 3") -> (x .or. y?=w1968:bool)
    "b" <- w1915
    "a" <- w1916
  }
  n74 = node-c288(w69) -> ()
  n75 = node-c288(w67) -> ()
  n76 = call-dynamic "Close Starter Kit.vi"("error in (no error)"=w37, "starter kit host in"=w38) -> ("error out"=w26:errorcluster)  [unwired: 9 in]
  n77 = call-dynamic "Close Starter Kit.vi"("error in (no error)"=w62, "starter kit host in"=w63) -> ("error out"=w51:errorcluster)  [unwired: 9 in]
  n78 = call <vilib>:"Stop Simulator Service.vi"("error in (no error)"=w26) -> ("error out"=w25:errorcluster)  [unwired: 10 in]
  n79 = call <vilib>:"Stop Simulator Service.vi"("error in (no error)"=w51) -> ("error out"=w50:errorcluster)  [unwired: 10 in]
  n80 = call <vilib>:"Simple Error Handler.vi"("error in (no error)"=w25) -> ()  [unwired: 4 in, 5 out]
  n81 = call <vilib>:"Simple Error Handler.vi"("error in (no error)"=w50) -> ()  [unwired: 4 in, 5 out]
